vi "Ocean Optics 2000 4000 Acquire Continuous Waveform.vi"() -> ()   [LabVIEW 2016]
doc: "Demonstrates continuous waveform measurement. Spectrum is displayed in a waveform graph."
uses:
  <vilib>/UPVI/lvhdf5/file.llb/LVH5F Operation.ctl
  <vilib>/UPVI/lvhdf5/dataset.llb/LVH5D Operation.ctl
  <vilib>/Utility/miscctls.llb/LVRectTypeDef.ctl
  <vilib>/UPVI/lvhdf5/group.llb/H5G_obj_t.ctl
  <vilib>/UPVI/lvhdf5/utility.llb/Select HDF5 Dialog.vi
  <vilib>/UPVI/lvhdf5/utility.llb/Select HDF5 Dialog (Object Only).vi
  <vilib>/UPVI/lvhdf5/dataset.llb/Simple H5Dwrite (Variant).vi
  <vilib>/UPVI/lvhdf5/dataset.llb/Simple H5Dwrite.xnode
  <vilib>/UPVI/lvhdf5/library.llb/HDF5 Ref.ctl
  <instrlib>/Ocean Optics 2000 4000/Ocean Optics 2000 4000.lvlib
  <vilib>/UPVI/lvhdf5/identifier.llb/Not an HDF5 Refnum Constant.vi
  <vilib>/Utility/error.llb/Error Cluster From Error Code.vi
  <vilib>/UPVI/lvhdf5/dataset.llb/OpenCreateReplace Dataset by Element Type.vi
  <vilib>/UPVI/lvhdf5/dataspace.llb/H5Sselect_hyperslab.vi
  <vilib>/UPVI/lvhdf5/dataset.llb/H5Dwrite (Variant).vi
  <vilib>/UPVI/lvhdf5/dataset.llb/H5Dget_space.vi
  <vilib>/UPVI/lvhdf5/attribute.llb/private/LVH5AwriteWDTAttrs.vi
  <vilib>/UPVI/lvhdf5/dataspace.llb/H5Sclose.vi
  <vilib>/UPVI/lvhdf5/dataset.llb/H5Dclose.vi
  <vilib>/UPVI/lvhdf5/utility.llb/Select HDF5 Dialog (File and Object).vi
panel:
  in  "Dataset Path":string
  in  "path":path
  in  "Boolean":bool
  in  "Number of Spectrum (5) 2":i32=5
  in  "Stop":bool
  out "Spectral Waveform":cluster{dbl[], dbl[]}(graph)
  in  "Enable Strobe (Disabled)":bool
  in  "VISA resource name":refnum<visa-resource-name>
  # "(c) 2009-2016 National Instruments.  ALL RIGHTS RESERVED."
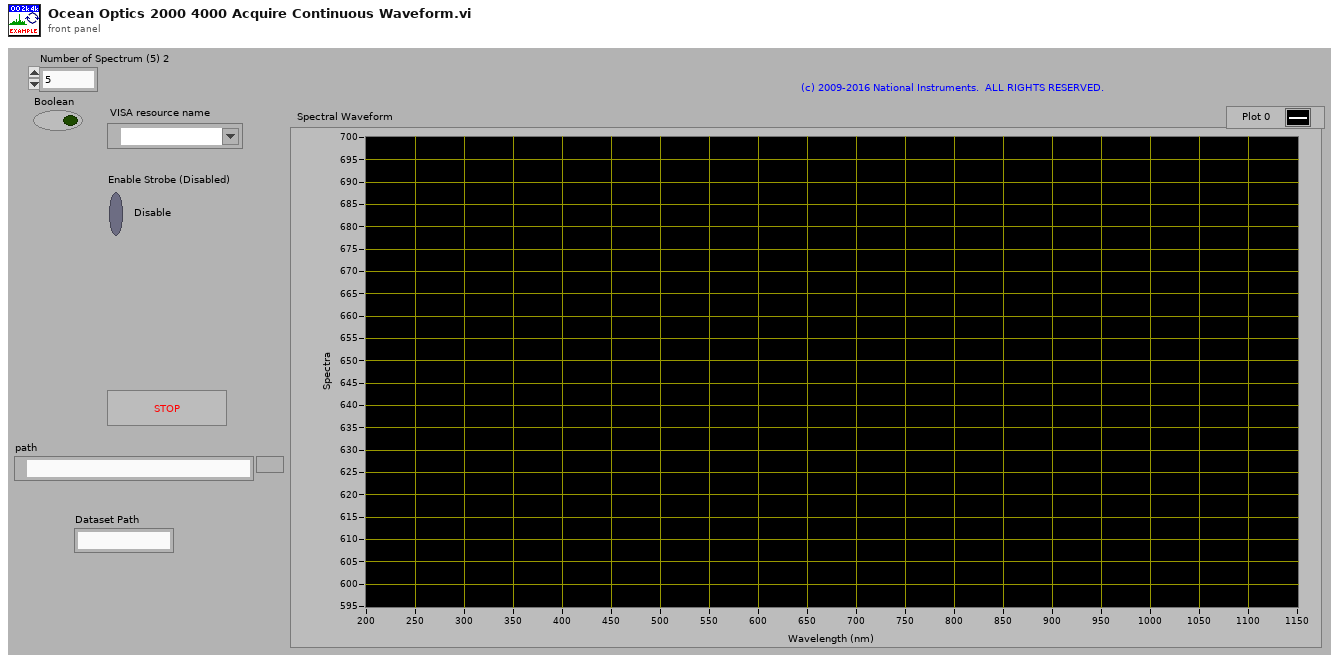
[diagram p1: front panel]
types:
  T1 = typedef "LVH5D Operation.ctl" = enum16{"open", "replace", "create", "open or create", "create or replace", "create or replace with confirmation"}
  T2 = typedef "LVH5F Operation.ctl" = enum16{"open", "open or create", "create or replace", "create or replace (with confirmation)", "create", "open (read only)"}
  T3 = typedef "LVRectTypeDef.ctl" = cluster{"Left":i16, "Top":i16, "Right":i16, "Bottom":i16}
  T4 = cluster{"Behavior":enum32{"Invalid", "Default", "Floating", "Floating/Auto-Hide", "Modal"}, "Position":T3, "Center":bool, "Title":string}
  T5 = typedef "H5G_obj_t.ctl" = i32
  T6 = cluster{"Object Types (any)":T5[], "Object Pattern":string}
  T7 = typedef "HDF5 Ref.ctl" = refnum<k1>
  T8 = cluster{"Wavelength (nm)":dbl[], "Spectrum by Pixel Number":dbl[]}
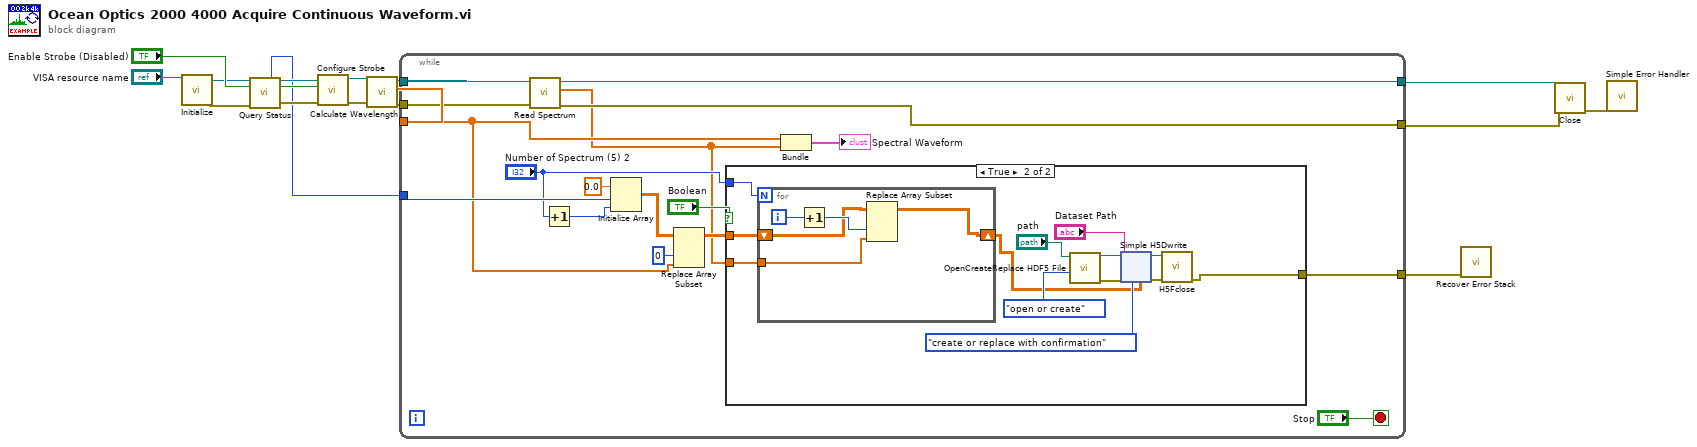
[diagram p0: block diagram]
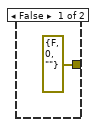
[diagram p2: hidden frame]
diagram:
  n1 = call <instrlib>:"Initialize.vi"("VISA resource name"="VISA resource name") -> ("error out"=w5:errorcluster, "VISA resource name out"=w6:refnum<visa-resource-name>)  [unwired: 2 in, 7 out]
  n2 = call <instrlib>:"Query Status.vi"("VISA resource name"=w6, "error in (no error)"=w5) -> ("Number of Pixels"=w2:u16, "VISA resource name out"=w4:refnum<visa-resource-name>, "error out"=w3:errorcluster)  [unwired: 11 out]
  n3 = call <instrlib>:"Configure Strobe.vi"("error in (no error)"=w3, "Enable Strobe (Disabled)"="Enable Strobe (Disabled)", "VISA resource name"=w4) -> ("error out"=w8:errorcluster, "VISA resource name out"=w9:refnum<visa-resource-name>)  [unwired: 7 out]
  n4 = call <instrlib>:"Calculate Wavelength.vi"("error in (no error)"=w8, "VISA resource name"=w9) -> ("error out"=w10:errorcluster, "Wavelength (nm)"=w12:dbl[], "VISA resource name out"=w11:refnum<visa-resource-name>)  [unwired: 1 in, 6 out]
  n5 = while {
    tunnel: [w32] -> w7
    tunnel: [w31] -> w15
    tunnel: w12 -> [w22]
    tunnel: w11 -> [w30]
    tunnel: w10 -> [w29]
    tunnel: w2 -> [w27]
    tunnel: [w17] -> w1
    stop <- "Stop" stop-if-true
    n6 = call <instrlib>:"Read Spectrum.vi"("error in (no error)"=w29, "VISA resource name"=w30) -> ("error out"=w31:errorcluster, "Spectrum by Pixel Number"=w18:dbl[], "VISA resource name out"=w32:refnum<visa-resource-name>)  [unwired: 6 in, 1 out]
    n7 = Increment(x="Number of Spectrum (5) 2") -> (x+1=w25:i32)
    n8 = Initialize Array(0.0 ("element"), w27, w25) -> (w23:dbl[][])
    n9 = Replace Array Subset(array=w23, new element=w22, index (col)=0) -> (w19:dbl[][])  [unwired: 1 in]
    n10 = case shown="True" "Boolean" {
      tunnel: "Number of Spectrum (5) 2" -> [_ w47]
      tunnel: w19 -> [_ w46]
      tunnel: w18 -> [_ w45]
      tunnel: [errorcluster {"status"=FALSE, "code"=0, "source"=""} ("error out") w35] -> w17
      frame False {
      }
      frame True {
        n11 = for {
          N: w47 -> [_]
          shift-right: [w251] -> w36
          shift-left: w46 -> [w252]
          tunnel: w45 -> [w250]
          i -> [w254]
          n12 = Increment(x=w254) -> (x+1=w253:i32)
          n13 = Replace Array Subset(array=w252, new element=w250, index (col)=w253) -> (w251:dbl[][])  [unwired: 1 in]
        }
        n14 = call <vilib>:"OpenCreateReplace HDF5 File.vi"("function (open or create)"=LVH5F_Operation."open or create", "path"="path") -> ("error out"=w42:errorcluster, "HDF5 Ref out"=w41:T7)  [unwired: 6 in]
        n15 = xnode "Simple H5Dwrite"("Dataset Path"="Dataset Path", "error in (no error)"=w42, "operation (open or create)"=LVH5D_Operation."create or replace with confirmation", "HDF5 Path or Ref"=w41, "Data"=w36) -> ("HDF5 Ref out"=w38:T7, "error out"=w39:errorcluster)  [unwired: 3 in, 1 out]
        n16 = call <vilib>:"H5Fclose.vi"("error in (no error)"=w39, "HDF5 Ref"=w38) -> ("error out"=w35:errorcluster)  [unwired: 7 in]
      }
    }
    n17 = Bundle("Wavelength (nm)"=w22, "Spectrum by Pixel Number"=w18) -> (→"Spectral Waveform":T8)  [unwired: 1 out]
  }
  n18 = call <vilib>:"Recover Error Stack.vi"("error in (no error)"=w1) -> ()  [unwired: 5 in, 4 out]
  n19 = call <instrlib>:"Close.vi"("error in (no error)"=w15, "VISA resource name"=w7) -> ("error out"=w14:errorcluster)  [unwired: 9 out]
  n20 = call <vilib>:"Simple Error Handler.vi"("error in (no error)"=w14) -> ()  [unwired: 1 in, 8 out]
